vi "ShieldSubVi_old.vi"(0 "DigNum Refnum":refnum<vi>, 1 "Str Refnum (Pos readout)":refnum<vi>, 2 "Bool Refnum (stop)":refnum<vi>, 3 "CmbBox Refnum":refnum<vi>, 4 "Bool Refnum (home)":refnum<vi>, 5 "Bool Refnum (power)":refnum<vi>, 6 "Bool Refnum (abort)":refnum<vi>, 7 "Bool Refnum (move)":refnum<vi>) -> ()   [LabVIEW 2014]
uses:
  <vilib>/Instr/_visa.llb/VISA Configure Serial Port (Instr).vi
  <vilib>/FieldPoint/Polymorphic Write.llb/FP Write (Boolean -IO).vi
panel:
  out "Shield Error":errorcluster caption="error out"
  out "Abort readout":string
  out "Home Readout":string
  in  "Move Stop Inner":bool
  in  "Steps 2":string(combo)
  out "Moving Readout 2":string
  out "Speed Readout 3":string
  out "Speed Readout 2":string
  out "Power":bool
  out "Numeric":i32
  out "Position Readout 2":string
  out "Position in Inches 2":ext format="%.4f"
  out "Position 2":ext(slide) scale=0.0..20.0 scale format="%#_2g"
  in  "Stop Position Reading":bool
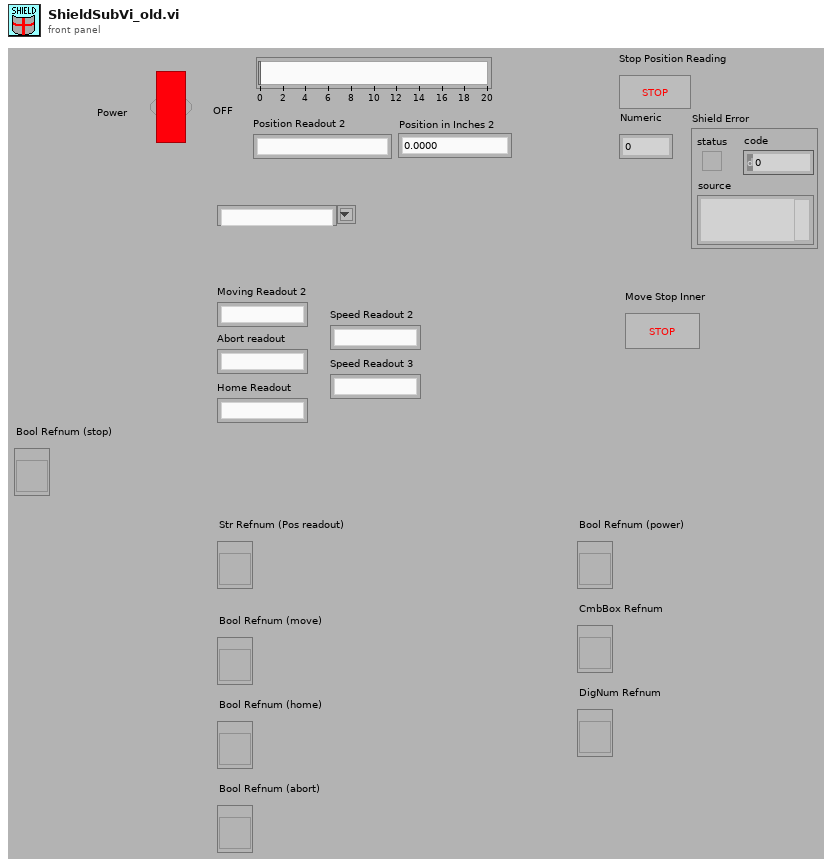
[diagram p1: front panel]
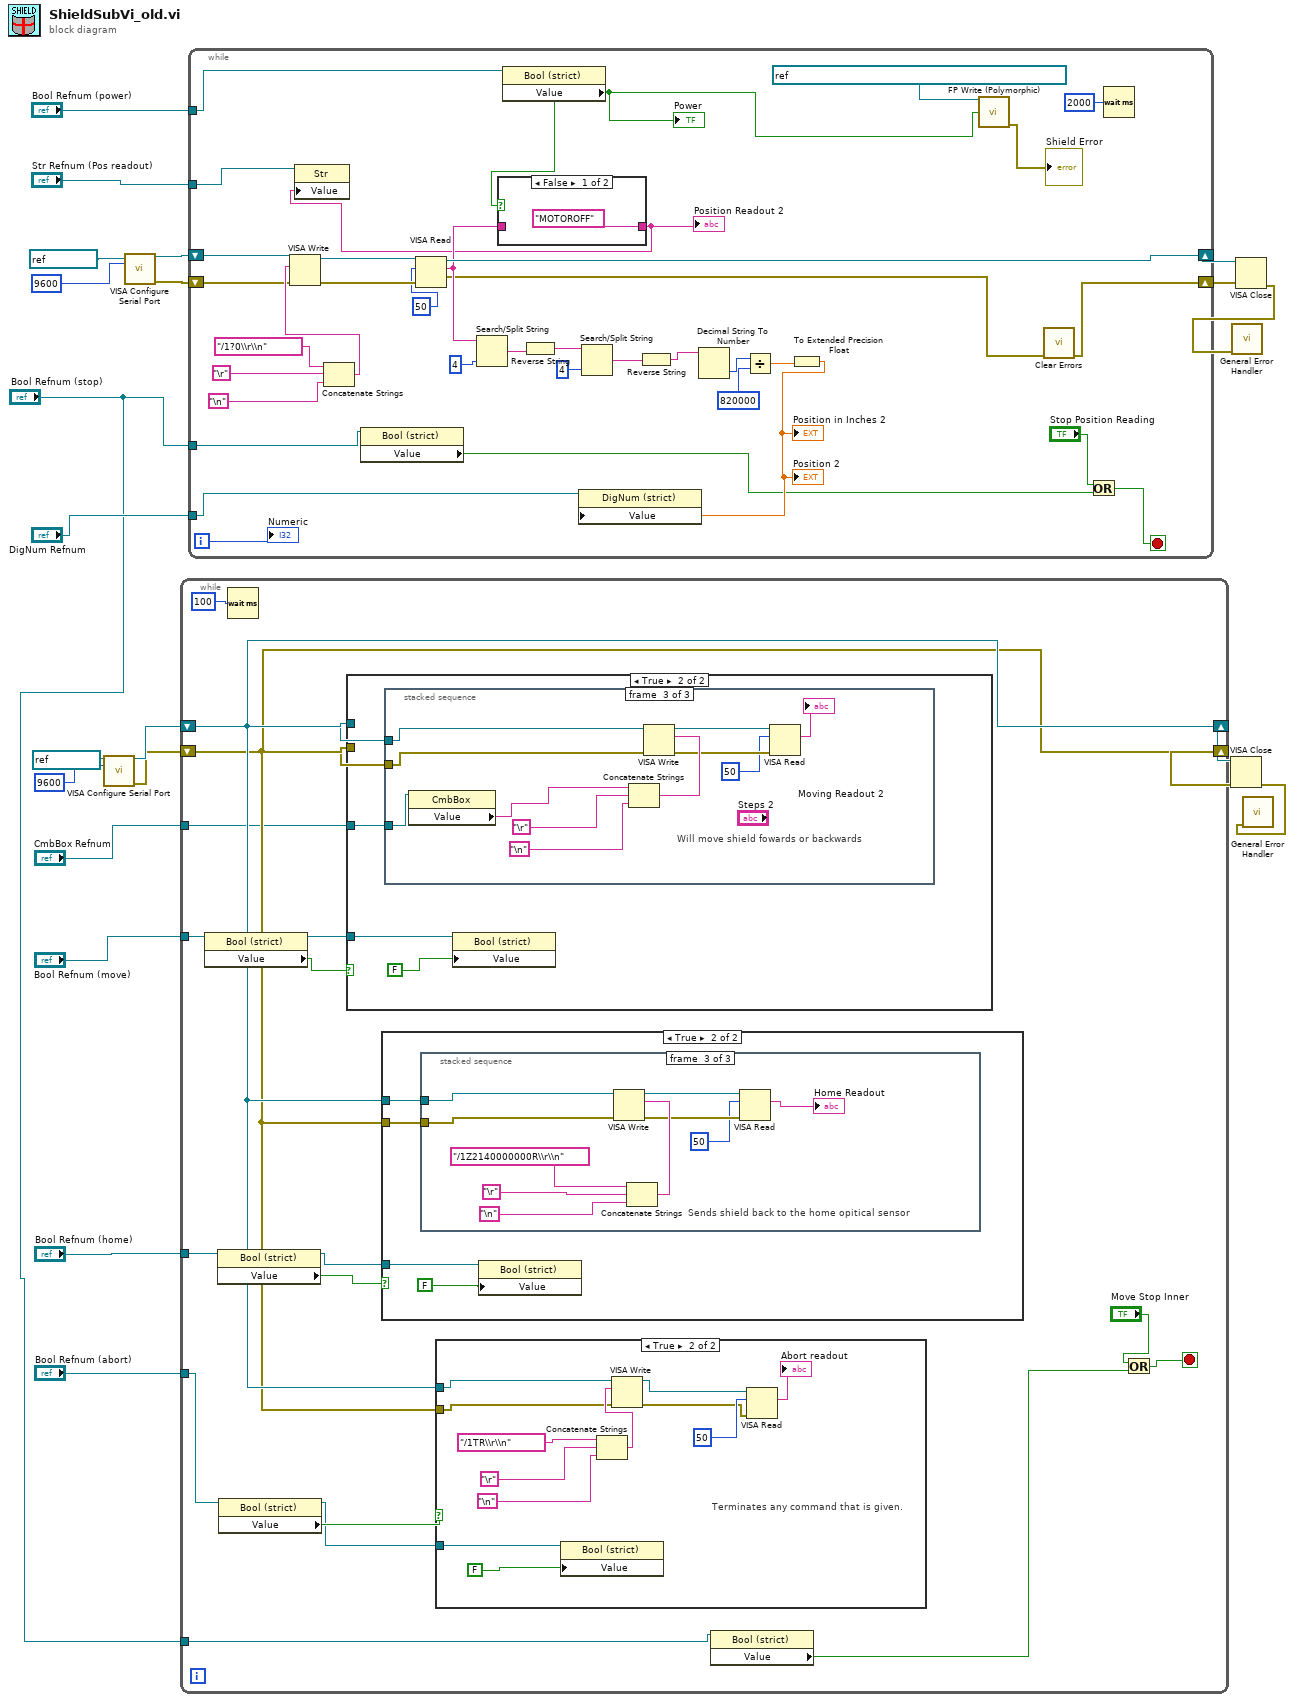
[diagram p0: block diagram]
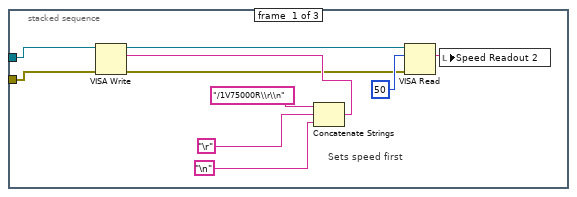
[diagram p5: hidden frame]
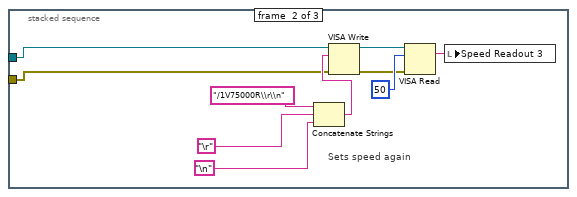
[diagram p6: hidden frame]
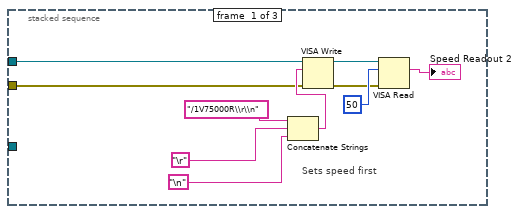
[diagram p8: hidden frame]
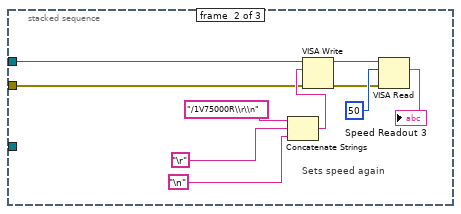
[diagram p9: hidden frame]
diagram:
  n1 = call-poly "VISA Configure Serial Port"("VISA resource name"=refnum<visa-resource-name> "COM30" ("Resource Name"), "baud rate (9600)"=u32 9600 ("Baud Rate (9600)")) -> ("VISA resource name out"=w22:refnum<visa-resource-name>, "error out"=w21:errorcluster)  [unwired: 12 in]
  n2 = call-poly "VISA Configure Serial Port"("VISA resource name"=refnum<visa-resource-name> "COM30" ("Resource Name"), "baud rate (9600)"=u32 9600 ("Baud Rate (9600)")) -> ("VISA resource name out"=w12:refnum<visa-resource-name>, "error out"=w13:errorcluster)  [unwired: 12 in]
  n3 = while {
    shift-right: [w38] -> w16
    shift-left: w22 -> [w38]
    shift-right: [w37] -> w17
    shift-left: w21 -> [w37]
    tunnel: "CmbBox Refnum" -> [w36]
    tunnel: "Bool Refnum (abort)" -> [w35]
    tunnel: "Bool Refnum (home)" -> [w33]
    tunnel: "Bool Refnum (move)" -> [w30]
    tunnel: "Bool Refnum (stop)" -> [w26]
    stop <- w25 stop-if-true
    n4 = property class="Bool (strict)"(reference=w30) -> (reference out=w29:refnum<vi>, "Value"=w28:bool)  [unwired: 1 in, 1 out]
    n5 = property class="Bool (strict)"(reference=w33) -> (reference out=w32:refnum<vi>, "Value"=w27:bool)  [unwired: 1 in, 1 out]
    n6 = property class="Bool (strict)"(reference=w35) -> (reference out=w31:refnum<vi>, "Value"=w34:bool)  [unwired: 1 in, 1 out]
    n7 = Wait (ms)(milliseconds to wait=u32 100) -> ()  [unwired: 1 out]
    n8 = case shown="True" w28 {
      tunnel: w38 -> [_ w90]
      tunnel: w37 -> [_ w89]
      tunnel: w36 -> [_ w88]
      tunnel: w29 -> [_ w87]
      frame False {
      }
      frame True {
        n9 = stacked-sequence {
          tunnel: w90 -> [w92 w102 w114]
          tunnel: w89 -> [w91 w101 w113]
          tunnel: w88 -> [_ _ w112]
          frame #0 {
            # "Sets speed first"
            n10 = Concatenate Strings("/1V75000R\\r\\n" ("string"), "\r", "\n") -> (w98:string)
            n11 = VISA Write(VISA resource name=w92, write buffer=w98, error in (no error)=w91) -> (VISA resource name out=w95:refnum<visa-resource-name>, error out=w94:errorcluster)  [unwired: 1 out]
            n12 = VISA Read(VISA resource name=w95, byte count=u32 50, error in (no error)=w94) -> (read buffer=→"Speed Readout 2":string)  [unwired: 3 out]
          }
          frame #1 {
            # "Sets speed again"
            n13 = Concatenate Strings("/1V75000R\\r\\n" ("string"), "\r", "\n") -> (w108:string)
            n14 = VISA Write(VISA resource name=w102, write buffer=w108, error in (no error)=w101) -> (VISA resource name out=w105:refnum<visa-resource-name>, error out=w104:errorcluster)  [unwired: 1 out]
            n15 = VISA Read(VISA resource name=w105, byte count=u32 50, error in (no error)=w104) -> (read buffer=→"Speed Readout 3":string)  [unwired: 3 out]
          }
          frame #2 {
            # "Will move shield fowards or backwards"
            n16 = property class="CmbBox"(reference=w112) -> ("Value"=w111:string)  [unwired: 1 in, 2 out]
            n17 = Concatenate Strings(w111, "\r", "\n") -> (w119:string)
            n18 = VISA Write(VISA resource name=w114, write buffer=w119, error in (no error)=w113) -> (VISA resource name out=w116:refnum<visa-resource-name>, error out=w117:errorcluster)  [unwired: 1 out]
            n19 = VISA Read(VISA resource name=w116, byte count=u32 50, error in (no error)=w117) -> (read buffer=→"Moving Readout 2":string)  [unwired: 3 out]
          }
        }
        n20 = property class="Bool (strict)"(reference=w87, "Value"=FALSE) -> ()  [unwired: 1 in, 2 out]
      }
    }
    n21 = case shown="True" w27 {
      tunnel: w38 -> [_ w55]
      tunnel: w37 -> [_ w54]
      tunnel: w32 -> [_ w53]
      frame False {
      }
      frame True {
        n22 = stacked-sequence {
          tunnel: w55 -> [w57 w67 w82]
          tunnel: w54 -> [w58 w68 w81]
          frame #0 {
            # "Sets speed first"
            n23 = Concatenate Strings("/1V75000R\\r\\n" ("string"), "\r", "\n") -> (w63:string)
            n24 = VISA Write(VISA resource name=w57, write buffer=w63, error in (no error)=w58) -> (VISA resource name out=w61:refnum<visa-resource-name>, error out=w60:errorcluster)  [unwired: 1 out]
            n25 = VISA Read(VISA resource name=w61, byte count=u32 50, error in (no error)=w60) -> (read buffer=w56:string)  [unwired: 3 out]
            n26 = local write "Speed Readout 2"(w56) -> ()
          }
          frame #1 {
            # "Sets speed again"
            n27 = Concatenate Strings("/1V75000R\\r\\n" ("string"), "\r", "\n") -> (w73:string)
            n28 = VISA Write(VISA resource name=w67, write buffer=w73, error in (no error)=w68) -> (VISA resource name out=w71:refnum<visa-resource-name>, error out=w70:errorcluster)  [unwired: 1 out]
            n29 = VISA Read(VISA resource name=w71, byte count=u32 50, error in (no error)=w70) -> (read buffer=w66:string)  [unwired: 3 out]
            n30 = local write "Speed Readout 3"(w66) -> ()
          }
          frame #2 {
            # "Sends shield back to the home opitical sensor"
            n31 = Concatenate Strings("/1Z2140000000R\\r\\n", "\r", "\n") -> (w83:string)
            n32 = VISA Write(VISA resource name=w82, write buffer=w83, error in (no error)=w81) -> (VISA resource name out=w78:refnum<visa-resource-name>, error out=w79:errorcluster)  [unwired: 1 out]
            n33 = VISA Read(VISA resource name=w78, byte count=u32 50, error in (no error)=w79) -> (read buffer=→"Home Readout":string)  [unwired: 3 out]
          }
        }
        n34 = property class="Bool (strict)"(reference=w53, "Value"=FALSE) -> ()  [unwired: 1 in, 2 out]
      }
    }
    n35 = case shown="True" w34 {
      tunnel: w38 -> [_ w48]
      tunnel: w37 -> [_ w47]
      tunnel: w31 -> [_ w40]
      frame False {
      }
      frame True {
        # "Terminates any command that is given."
        n36 = property class="Bool (strict)"(reference=w40, "Value"=FALSE) -> ()  [unwired: 1 in, 2 out]
        n37 = Concatenate Strings("/1TR\\r\\n", "\r", "\n") -> (w49:string)
        n38 = VISA Write(VISA resource name=w48, write buffer=w49, error in (no error)=w47) -> (VISA resource name out=w43:refnum<visa-resource-name>, error out=w42:errorcluster)  [unwired: 1 out]
        n39 = VISA Read(VISA resource name=w43, byte count=u32 50, error in (no error)=w42) -> (read buffer=→"Abort readout":string)  [unwired: 3 out]
      }
    }
    n40 = property class="Bool (strict)"(reference=w26) -> ("Value"=w23:bool)  [unwired: 1 in, 2 out]
    n41 = Or(x="Move Stop Inner", y=w23) -> (x .or. y?=w25:bool)
  }
  n42 = while {
    shift-right: [w138] -> w11
    shift-left: w12 -> [w140]
    shift-right: [w136] -> w10
    shift-left: w13 -> [w139]
    tunnel: "Str Refnum (Pos readout)" -> [w133]
    tunnel: "Bool Refnum (power)" -> [w131]
    tunnel: "DigNum Refnum" -> [w129]
    tunnel: "Bool Refnum (stop)" -> [w125]
    i -> [w157]
    stop <- w122 stop-if-true
    n43 = Concatenate Strings("/1?0\\r\\n", "\r", "\n") -> (w153:string)
    n44 = VISA Write(VISA resource name=w140, write buffer=w153, error in (no error)=w139) -> (VISA resource name out=w155:refnum<visa-resource-name>, error out=w156:errorcluster)  [unwired: 1 out]
    n45 = property class="Bool (strict)"(reference=w125) -> ("Value"=w123:bool)  [unwired: 1 in, 2 out]
    n46 = VISA Read(VISA resource name=w155, byte count=u32 50, error in (no error)=w156) -> (VISA resource name out=w138:refnum<visa-resource-name>, read buffer=w135:string, error out=w134:errorcluster)  [unwired: 1 out]
    n47 = Search/Split String(string=w135, offset (0)=4) -> (match + rest of string=w143:string)  [unwired: 1 in, 2 out]
    n48 = property class="Bool (strict)"(reference=w131) -> ("Value"=w127:bool)  [unwired: 1 in, 2 out]
    "Power" <- w127
    n49 = case shown="False" w127 {
      tunnel: w135 -> [_ w159]
      tunnel: ["MOTOROFF" w159] -> w132
      frame False {
      }
      frame True {
      }
    }
    "Position Readout 2" <- w132
    n50 = property class="Str"(reference=w133, "Value"=w132) -> ()  [unwired: 1 in, 2 out]
    n51 = Reverse String(1:w143) -> (0:w144:string)
    n52 = Search/Split String(string=w144, offset (0)=4 ("offset (0) 2")) -> (match + rest of string=w145:string)  [unwired: 1 in, 2 out]
    n53 = Reverse String(1:w145) -> (0:w146:string)
    n54 = Decimal String To Number(string=w146) -> (number=w147:i32)  [unwired: 2 in, 1 out]
    n55 = Divide(x=w147, y=820000) -> (x/y=w148:dbl)
    n56 = To Extended Precision Float(1:w148) -> (0:w130:ext)
    "Position in Inches 2" <- w130
    "Position 2" <- w130
    n57 = property class="DigNum (strict)"(reference=w129, "Value"=w130) -> ()  [unwired: 1 in, 2 out]
    n58 = call-poly <vilib>:"FP Write (Polymorphic).vi"("FieldPoint IO Point In"=refnum<k21> "FieldPoint\\FP @ COM33\\FP-DIO-550 @2\\Output 3" ("FieldPoint IO Point"), "value"=w127) -> ("error out"=→"Shield Error":errorcluster)  [unwired: 11 in, 2 out]
    n59 = call <vilib>:"Clear Errors.vi"("error in (no error)"=w134) -> ("error out"=w136:errorcluster)  [unwired: 5 in, 1 out]
    n60 = Or(x="Stop Position Reading", y=w123) -> (x .or. y?=w122:bool)
    n61 = Wait (ms)(milliseconds to wait=u32 2000) -> ()  [unwired: 1 out]
    "Numeric" <- w157
  }
  n62 = VISA Close(VISA resource name=w16, error in (no error)=w17) -> (error out=w18:errorcluster)
  n63 = VISA Close(VISA resource name=w11, error in (no error)=w10) -> (error out=w9:errorcluster)
  n64 = call <vilib>:"General Error Handler.vi"("error in (no error)"=w9) -> ()  [unwired: 10 in, 5 out]
  n65 = call <vilib>:"General Error Handler.vi"("error in (no error)"=w18) -> ()  [unwired: 10 in, 5 out]
